vi "ShooterStateController.vi"(1 "Selected State (In)":string) -> (0 "Selected State (Out)":string)   [LabVIEW 2019]
doc: "This VI makes all calculations and decisions related to the shooter subsystem."
uses:
  dsinstructions.vi
  sensors.vi
  constants.vi
  dsdata.vi
  outputs.vi
panel:
  in  "Cowl_Position_Offset":dbl
  in  "Cowl Position Error Threshold (a)":dbl
  in  "Cowl_Position_(a)":dbl
  in  "Far_Trench_Angle (a)":dbl
  in  "Close_Trench_Angle (a)":dbl
  in  "Initiation_Line_Angle (a)":dbl
  in  "Wall_Angle (a)":dbl
  out "Goal_Cowl_Position_(a)":dbl
  in  "Shooter Prespin (ms)":u32=7000
  in  "Settling Time (ms)":u32=500
  in  "Shooter Off Delay (ms)":u32=1000
  in  "Max Range (in)":dbl=1000.0
  in  "Max Acceptable Robot Speed (ft/s)":dbl=5.0
  in  "Acceptable Shooter Error Fraction":dbl=0.1
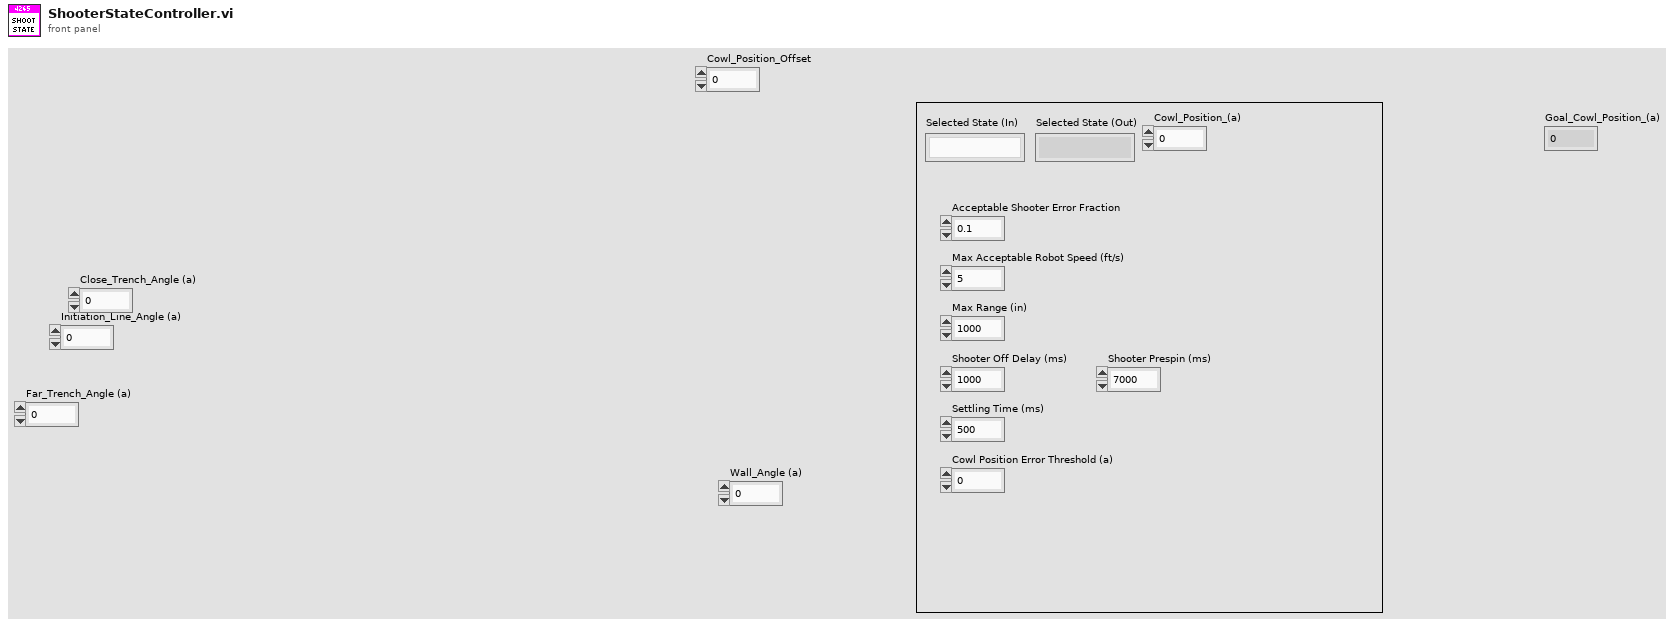
[diagram p1: front panel]
types:
  T1 = enum16{"Center", "North", "NorthWest", "West", "SouthWest", "South", "SouthEast", "East", "NorthEast"}
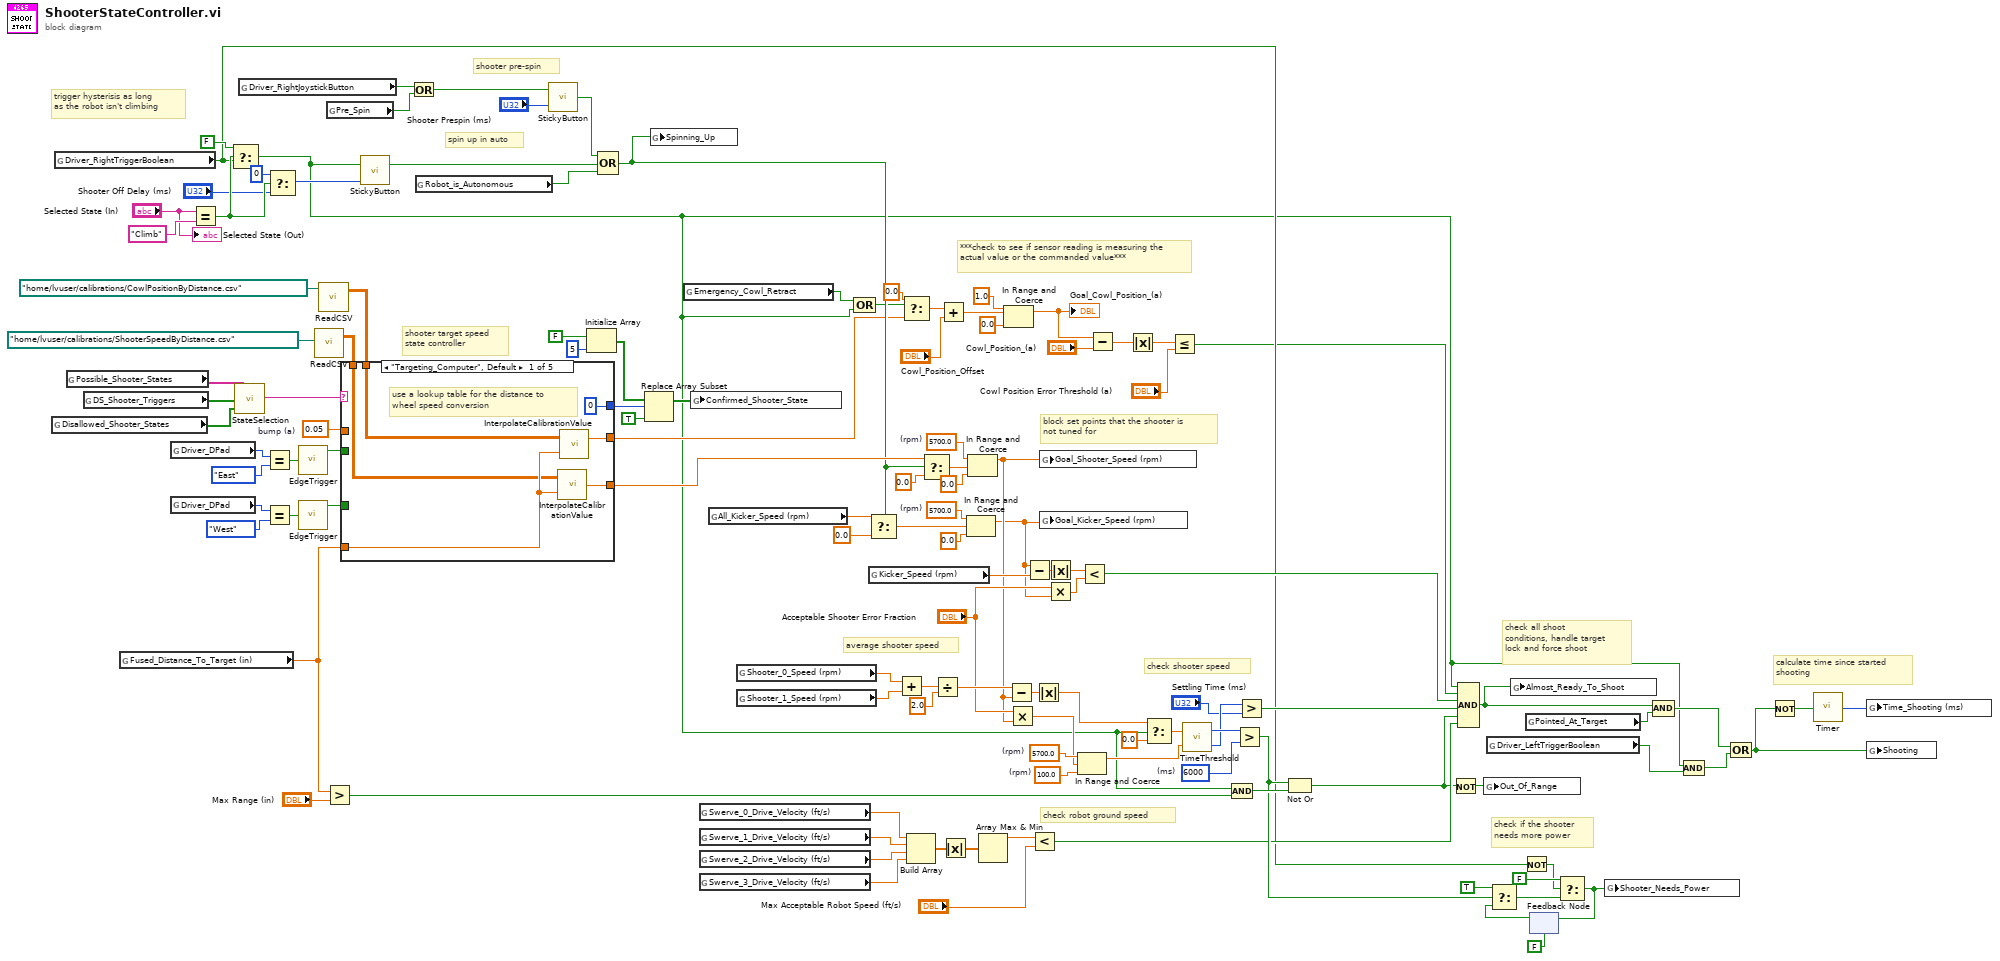
[diagram p0: block diagram]
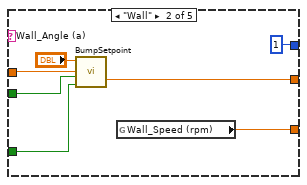
[diagram p2: hidden frame]
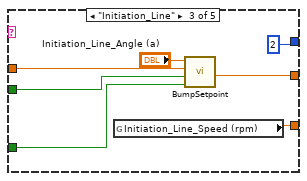
[diagram p3: hidden frame]
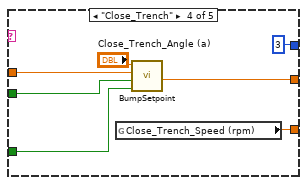
[diagram p4: hidden frame]
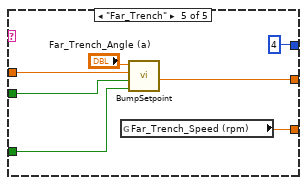
[diagram p5: hidden frame]
diagram:
  w30 = 0.05  # bump (a)
  w76 = 100.0  # (rpm)
  w77 = 5700.0  # (rpm)
  w85 = 5700.0  # (rpm)
  w89 = 5700.0  # (rpm)
  w95 = u32 6000  # (ms)
  # "***check to see if sensor reading is measuring the actual value or the commanded value***"
  # "calculate time since started\nshooting"
  # "check if the shooter\nneeds more power"
  # "average shooter speed"
  # "check shooter speed"
  # "shooter target speed\nstate controller"
  # "shooter pre-spin"
  # "check all shoot\nconditions, handle target\nlock and force shoot"
  # "spin up in auto"
  # "trigger hysterisis as long\nas the robot isn't climbing"
  # "check robot ground speed"
  # "block set points that the shooter is \nnot tuned for"
  n1 = global read "outputs.vi" "Disallowed_Shooter_States"() -> (w24:bool[])
  n2 = global read "dsinstructions.vi" "Driver_RightTriggerBoolean"() -> (w29:bool)
  n3 = global read "constants.vi" "Possible_Shooter_States"() -> (w114:string[])
  n4 = global read "dsinstructions.vi" "DS_Shooter_Triggers"() -> (w113:bool[])
  n5 = global read "sensors.vi" "Fused_Distance_To_Target (in)"() -> (w91:dbl)
  n6 = global read "dsinstructions.vi" "Driver_DPad"() -> (w50:T1)
  n7 = global read "dsinstructions.vi" "Driver_DPad"() -> (w46:T1)
  n8 = Equal?(x="Selected State (In)", y="Climb") -> (x = y?=w64:bool)
  n9 = Select(t=FALSE, s=w64, f=w29) -> (s? t:f=w12:bool)
  n10 = call "StateSelection.vi"("Disallowed States"=w24, "State Triggers"=w113, "State Names"=w114) -> ("Selected State"=w92:string)
  n11 = global read "dsinstructions.vi" "Driver_RightJoystickButton"() -> (w41:bool)
  n12 = Equal?(x=w50, y=T1."East" ("Driver_DPad")) -> (x = y?=w48:bool)
  n13 = Equal?(x=w46, y=T1."West" ("Driver_DPad")) -> (x = y?=w45:bool)
  n14 = Select(t=u32 0, s=w64, f="Shooter Off Delay (ms)") -> (s? t:f=w20:u32)
  n15 = call "EdgeTrigger.vi"("Input Signal"=w48) -> ("Rising Edge Trigger"=w47:bool)  [unwired: 2 out]
  n16 = call "EdgeTrigger.vi"("Input Signal"=w45) -> ("Rising Edge Trigger"=w43:bool)  [unwired: 2 out]
  n17 = call "ReadCSV.vi"("File Path (.csv)"=path "/home/lvuser/calibrations/ShooterSpeedByDistance.csv" ("path")) -> ("Data (index by row)"=w17:dbl[][])  [unwired: 1 in, 1 out]
  n18 = call "ReadCSV.vi"("File Path (.csv)"=path "/home/lvuser/calibrations/CowlPositionByDistance.csv" ("path")) -> ("Data (index by row)"=w18:dbl[][])  [unwired: 1 in, 1 out]
  n19 = Greater?(x=w91, y="Max Range (in)") -> (0:w68:bool)
  n20 = global read "dsinstructions.vi" "Pre_Spin"() -> (w42:bool)
  n21 = case shown="\"Targeting_Computer\", Default" w92 {
    tunnel: [w127 w134 w141 w148 w155] -> w112
    tunnel: [0 1 2 3 4] -> w106
    tunnel: w91 -> [w126 _ _ _ _]
    tunnel: w47 -> [_ w131 w138 w145 w152]
    tunnel: w43 -> [_ w130 w137 w144 w151]
    tunnel: w30 -> [_ w132 w139 w146 w153]
    tunnel: w18 -> [w123 _ _ _ _]
    tunnel: w17 -> [w124 _ _ _ _]
    tunnel: [w125 w129 w136 w143 w150] -> w16
    frame "Targeting_Computer", Default {
      # "use a lookup table for the distance to\nwheel speed conversion"
      n22 = call "InterpolateCalibrationValue.vi"("Input"=w126, "Calibration Data"=w124) -> ("Interpolated Output"=w127:dbl)
      n23 = call "InterpolateCalibrationValue.vi"("Input"=w126, "Calibration Data"=w123) -> ("Interpolated Output"=w125:dbl)
    }
    frame "Wall" {
      n24 = call "BumpSetpoint.vi"("Bump Down Trigger"=w130, "Bump Up Trigger"=w131, "Bump Increment"=w132, "Original Setpoint"="Wall_Angle (a)") -> ("Bumped Setpoint"=w129:dbl)  [unwired: 7 in]
      n25 = global read "dsdata.vi" "Wall_Speed (rpm)"() -> (w134:dbl)
    }
    frame "Initiation_Line" {
      n26 = global read "dsdata.vi" "Initiation_Line_Speed (rpm)"() -> (w141:dbl)
      n27 = call "BumpSetpoint.vi"("Bump Down Trigger"=w137, "Bump Up Trigger"=w138, "Bump Increment"=w139, "Original Setpoint"="Initiation_Line_Angle (a)") -> ("Bumped Setpoint"=w136:dbl)  [unwired: 7 in]
    }
    frame "Close_Trench" {
      n28 = global read "dsdata.vi" "Close_Trench_Speed (rpm)"() -> (w148:dbl)
      n29 = call "BumpSetpoint.vi"("Bump Down Trigger"=w144, "Bump Up Trigger"=w145, "Bump Increment"=w146, "Original Setpoint"="Close_Trench_Angle (a)") -> ("Bumped Setpoint"=w143:dbl)  [unwired: 7 in]
    }
    frame "Far_Trench" {
      n30 = global read "dsdata.vi" "Far_Trench_Speed (rpm)"() -> (w155:dbl)
      n31 = call "BumpSetpoint.vi"("Bump Down Trigger"=w151, "Bump Up Trigger"=w152, "Bump Increment"=w153, "Original Setpoint"="Far_Trench_Angle (a)") -> ("Bumped Setpoint"=w150:dbl)  [unwired: 7 in]
    }
  }
  n32 = call "StickyButton.vi"("Time threshold (ms)"=w20, "Button Input"=w12) -> ("Sticky Button"=w19:bool)
  n33 = Or(x=w41, y=w42) -> (x .or. y?=w23:bool)
  n34 = global read "dsdata.vi" "Robot_is_Autonomous"() -> (w25:bool)
  n35 = call "StickyButton.vi"("Time threshold (ms)"="Shooter Prespin (ms)", "Button Input"=w23) -> ("Sticky Button"=w21:bool)
  n36 = Initialize Array(FALSE, 5 ("dimension size")) -> (w109:bool[])
  n37 = Compound Arithmetic op=OR(w21, w19, w25) -> (w40:bool)
  n38 = Replace Array Subset(array=w109, new element=TRUE ("new element/subarray"), index=w106) -> (w107:bool[])
  n39 = global write "outputs.vi" "Spinning_Up"(w40) -> ()
  n40 = global read "dsdata.vi" "Emergency_Cowl_Retract"() -> (w13:bool)
  n41 = global write "outputs.vi" "Confirmed_Shooter_State"(w107) -> ()
  n42 = global read "sensors.vi" "Swerve_0_Drive_Velocity (ft/s)"() -> (w105:dbl)
  n43 = global read "sensors.vi" "Swerve_1_Drive_Velocity (ft/s)"() -> (w104:dbl)
  n44 = global read "sensors.vi" "Swerve_2_Drive_Velocity (ft/s)"() -> (w103:dbl)
  n45 = global read "sensors.vi" "Swerve_3_Drive_Velocity (ft/s)"() -> (w102:dbl)
  n46 = global read "dsdata.vi" "All_Kicker_Speed (rpm)"() -> (w83:dbl)
  n47 = global read "sensors.vi" "Shooter_0_Speed (rpm)"() -> (w120:dbl)
  n48 = global read "sensors.vi" "Shooter_1_Speed (rpm)"() -> (w119:dbl)
  n49 = Compound Arithmetic op=OR(w13, w12) -> (w11:bool)
  n50 = Select(t=w83, s=w40, f=0.0) -> (s? t:f=w82:dbl)
  n51 = global read "sensors.vi" "Kicker_Speed (rpm)"() -> (w81:dbl)
  n52 = Add(x=w120, y=w119) -> (x+y=w118:dbl)
  n53 = Select(t=0.0, s=w11, f=w16) -> (s? t:f=w3:dbl)
  n54 = Build Array(w105, w104, w103, w102) -> (w101:dbl[])
  n55 = Select(t=w112, s=w40, f=0.0) -> (s? t:f=w90:dbl)
  n56 = Divide(x=w118, y=2.0) -> (x/y=w115:dbl)
  n57 = Add(x=w3, y="Cowl_Position_Offset") -> (x+y=w2:dbl)
  n58 = Absolute Value(x=w101) -> (abs(x)=w100:dbl[])
  n59 = In Range and Coerce(upper limit=w85, x=w82, lower limit=0.0) -> (coerced(x)=w39:dbl)  [unwired: 1 out]
  n60 = In Range and Coerce(upper limit=w89, x=w90, lower limit=0.0) -> (coerced(x)=w72:dbl)  [unwired: 1 out]
  n61 = Array Max & Min(array=w100) -> (max value=w99:dbl)  [unwired: 3 out]
  n62 = In Range and Coerce(upper limit=1.0, x=w2, lower limit=0.0) -> (coerced(x)=w9:dbl)  [unwired: 1 out]
  "Goal_Cowl_Position_(a)" <- w9
  n63 = Subtract(x=w115, y=w72) -> (x-y=w116:dbl)
  n64 = Multiply(x="Acceptable Shooter Error Fraction", y=w72) -> (x*y=w75:dbl)
  n65 = Subtract(x=w39, y=w81) -> (x-y=w80:dbl)
  n66 = Less?(x=w99, y="Max Acceptable Robot Speed (ft/s)") -> (x < y?=w38:bool)
  n67 = Absolute Value(x=w116) -> (abs(x)=w71:dbl)
  n68 = global write "outputs.vi" "Goal_Shooter_Speed (rpm)"(w72) -> ()
  n69 = global write "outputs.vi" "Goal_Kicker_Speed (rpm)"(w39) -> ()
  n70 = Absolute Value(x=w80) -> (abs(x)=w73:dbl)
  n71 = Multiply(x="Acceptable Shooter Error Fraction", y=w39) -> (x*y=w78:dbl)
  n72 = In Range and Coerce(upper limit=w77, x=w75, lower limit=w76) -> (coerced(x)=w74:dbl)  [unwired: 1 out]
  n73 = Less?(x=w73, y=w78) -> (x < y?=w34:bool)
  n74 = Subtract(x=w9, y="Cowl_Position_(a)") -> (x-y=w7:dbl)
  n75 = Absolute Value(x=w7) -> (abs(x)=w6:dbl)
  n76 = Select(t=w71, s=w12, f=0.0) -> (s? t:f=w70:dbl)
  n77 = Less Or Equal?(x=w6, y="Cowl Position Error Threshold (a)") -> (x <= y?=w4:bool)
  n78 = call "TimeThreshold.vi"("Threshold"=w74, "Current Value"=w70) -> ("Time Below Threshold (ms)"=w52:u32, "Time Above Threshold (ms)"=w96:u32)
  n79 = And(x=w12, y=w68) -> (x .and. y?=w67:bool)
  n80 = Greater?(x=w96, y=w95) -> (0:w60:bool)
  n81 = Greater?(x=w52, y="Settling Time (ms)") -> (0:w35:bool)
  n82 = Not Or(1:w67, 2:w60) -> (0:w36:bool)
  n83 = Not(x=w36) -> (.not. x?=w37:bool)
  n84 = Compound Arithmetic op=AND(w12, w4, w34, w35, w36, w38) -> (w33:bool)
  n85 = global write "outputs.vi" "Out_Of_Range"(w37) -> ()
  n86 = global read "dsinstructions.vi" "Driver_LeftTriggerBoolean"() -> (w32:bool)
  n87 = global write "outputs.vi" "Almost_Ready_To_Shoot"(w33) -> ()
  n88 = Not(x=w29) -> (.not. x?=w53:bool)
  n89 = global read "sensors.vi" "Pointed_At_Target"() -> (w87:bool)
  n90 = feedback #1(FALSE) -> (w58:bool)
  n91 = Select(t=TRUE, s=w60, f=w58) -> (s? t:f=w56:bool)
  n92 = Select(t=FALSE, s=w53, f=w56) -> (s? t:f=w54:bool)
  n93 = feedback-in #1(w54) -> ()
  n94 = global write "outputs.vi" "Shooter_Needs_Power"(w54) -> ()
  n95 = Compound Arithmetic op=AND(w33, w87) -> (w88:bool)
  n96 = Compound Arithmetic op=AND(w12, w32) -> (w31:bool)
  n97 = Compound Arithmetic op=OR(w88, w31) -> (w28:bool)
  n98 = Not(x=w28) -> (.not. x?=w27:bool)
  n99 = call "Timer.vi"("Reset Timer"=w27) -> ("Time (ms)"=w26:u32)
  n100 = global write "outputs.vi" "Time_Shooting (ms)"(w26) -> ()
  n101 = global write "outputs.vi" "Shooting"(w28) -> ()
  "Selected State (Out)" <- "Selected State (In)"
